vi "tx metadata make.vi"(5 "end_of_burst":i32, 6 "start_of_burst":i32, 7 "frac_secs":dbl, 8 "error in (no error)":errorcluster, 9 "full_secs":i64, 10 "has_time_spec":i32, 11 "handle":u64) -> (0 "error out":errorcluster, 2 "function return":u32(ring), 3 "handle out":u64)   [LabVIEW 2024, in "uhd.lvlib"]
doc: "UHD_API uhd_error uhd_tx_metadata_make(uhd_tx_metadata_handle* handle,\n bool has_time_spec,\n int64_t full_secs,\n double frac_secs,\n bool start_of_burst,\n bool end_of_burst);"
uses:
  uhd.lvlib
  uhd.so
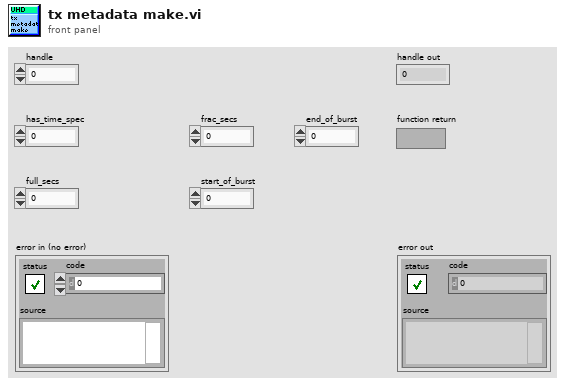
[diagram p1: front panel]
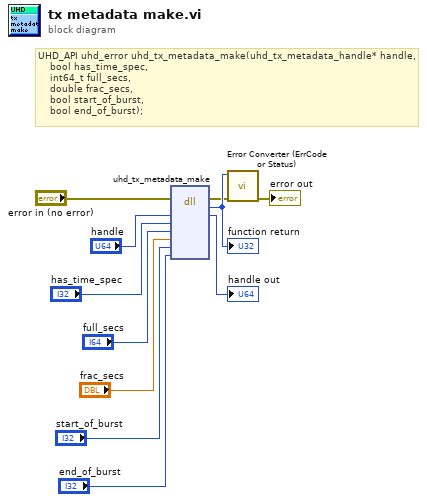
[diagram p0: block diagram]
diagram:
  # "UHD_API uhd_error uhd_tx_metadata_make(uhd_tx_metadata_handle* handle,\n    bool has_time_spec,\n    int64_t full_secs,\n    double frac_secs,\n    bool start_of_burst,\n    bool end_of_burst);"
  n1 = dll-call lib="uhd.*" fn="uhd_tx_metadata_make"(error in="error in (no error)", "handle"="handle", "has_time_spec"="has_time_spec", "full_secs"="full_secs", "frac_secs"="frac_secs", "start_of_burst"="start_of_burst", "end_of_burst"="end_of_burst") -> (error out=w2:errorcluster, w11:u32, "handle"=→"handle out":u64)  [unwired: 7 in, 1 out]
  "function return" <- w11
  n2 = call "Error Converter (ErrCode or Status).vi"("error in (no error)"=w2, "error code"=w11) -> ("error out"=→"error out":errorcluster)  [unwired: 9 in]
